vi "Get Power Meter.vi"(11 "error in (no error)":errorcluster) -> (4 "Power Meter Base out":refnum<class "Power Meter Base.lvclass">, 15 "error out":errorcluster)   [LabVIEW 2023, in "RFFixtureCharact.Instruments.lvlib" / "Power Meter Factory.lvclass"]
uses:
  Power Meter Factory.lvclass
  Power Meter Base/Power Meter Base.lvclass
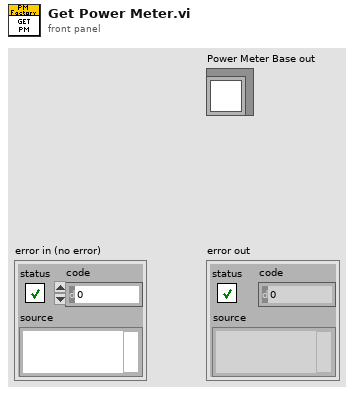
[diagram p1: front panel]
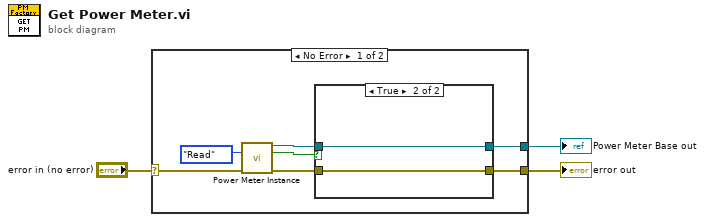
[diagram p0: block diagram]
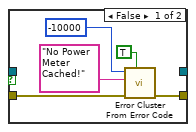
[diagram p2: hidden frame]
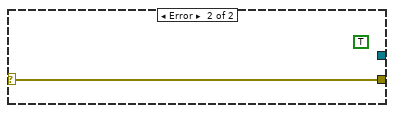
[diagram p3: hidden frame]
diagram:
  n1 = case shown="No Error" "error in (no error)" {
    selector: "error in (no error)" -> [w8 w18]
    tunnel: [w7 w18] -> w2
    tunnel: [w6 _] -> w1
    frame No Error {
      n2 = call "Power Meter Instance.vi"("Operation"=enum16{"Read", "Write", "Clear"}."Read", "error in (no error)"=w8) -> ("Power Meter out"=w10:refnum<class "Power Meter Base.lvclass">, "Found?"=w5:bool, "error out"=w9:errorcluster)  [unwired: 11 in]
      n3 = case shown="True" w5 {
        tunnel: w10 -> [_ w17]
        tunnel: w9 -> [w12 w16]
        tunnel: [w11 w16] -> w7
        tunnel: [_ w17] -> w6
        frame False {
          n4 = call <vilib>:"Error Cluster From Error Code.vi"("show call chain? (False)"=TRUE, "error in (no error)"=w12, "error message (\"\")"="No Power Meter Cached!" ("error message (\"\")"), "error code (0)"=-10000) -> ("error out"=w11:errorcluster)  [unwired: 5 in]
        }
        frame True {
        }
      }
    }
    frame Error {
      (unwired) TRUE
    }
  }
  "error out" <- w2
  "Power Meter Base out" <- w1
